vi "Is Connected.vi"(8 "error in (no error)":errorcluster, 11 "session in":refnum<class "Session.lvclass">) -> (0 "error out":errorcluster, 2 "is connected?":bool, 3 "session out":refnum<class "Session.lvclass">)   [LabVIEW 2020, in "NI_SFTP.lvlib" / "Session.lvclass"]
uses:
  <vilib>/net/SFTP/Session/Session.lvclass
  <vilib>/net/SFTP/Session/Session.lvclass/Session.ctl
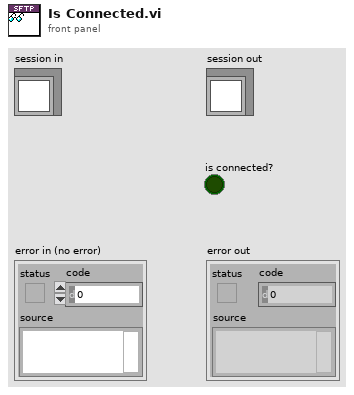
[diagram p1: front panel]
types:
  T1 = typedef "Semaphore RefNum" = refnum<k1>
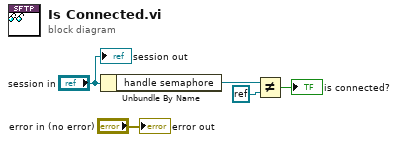
[diagram p0: block diagram]
diagram:
  n1 = Unbundle By Name("session in") -> ("handle semaphore"=w3:T1)
  n2 = Not Equal?(x=w3, y=refnum<k0> refnum) -> (x != y?=→"is connected?":bool)
  "error out" <- "error in (no error)"
  "session out" <- "session in"
